vi "Esercitazione 4 - Incertezza di categoria A.vi"() -> ()   [LabVIEW 2021]
panel:
  out "Relative uncertainty value (%)":dbl
  out "Absolute uncertainty":dbl format="%#_6f"
  out "Experimental waste":dbl format="%#_6f"
  out "Array":dbl[](array[numeric])
  out "Best estimate of the measurand":dbl
  out "sum":dbl
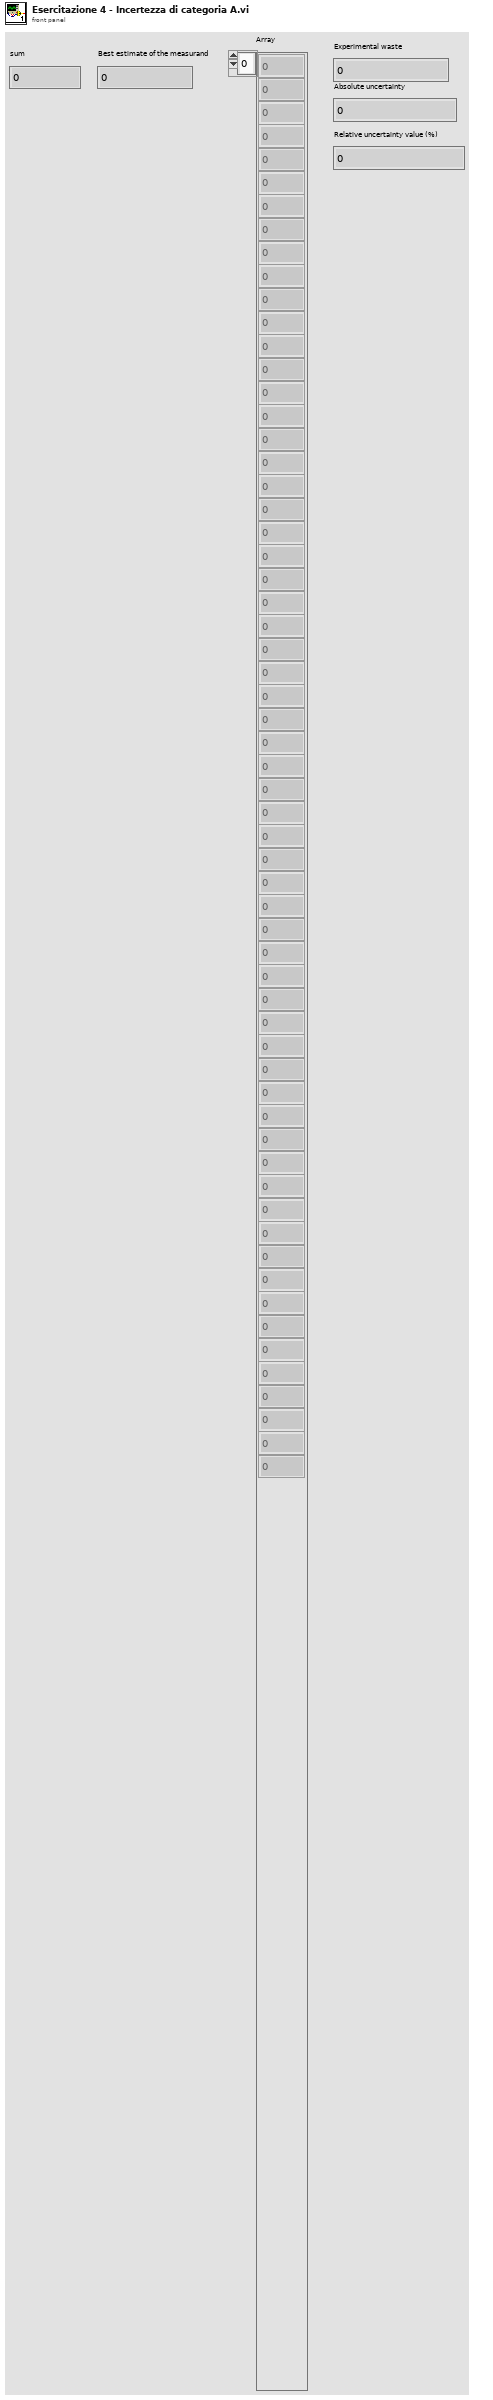
[diagram p1: front panel]
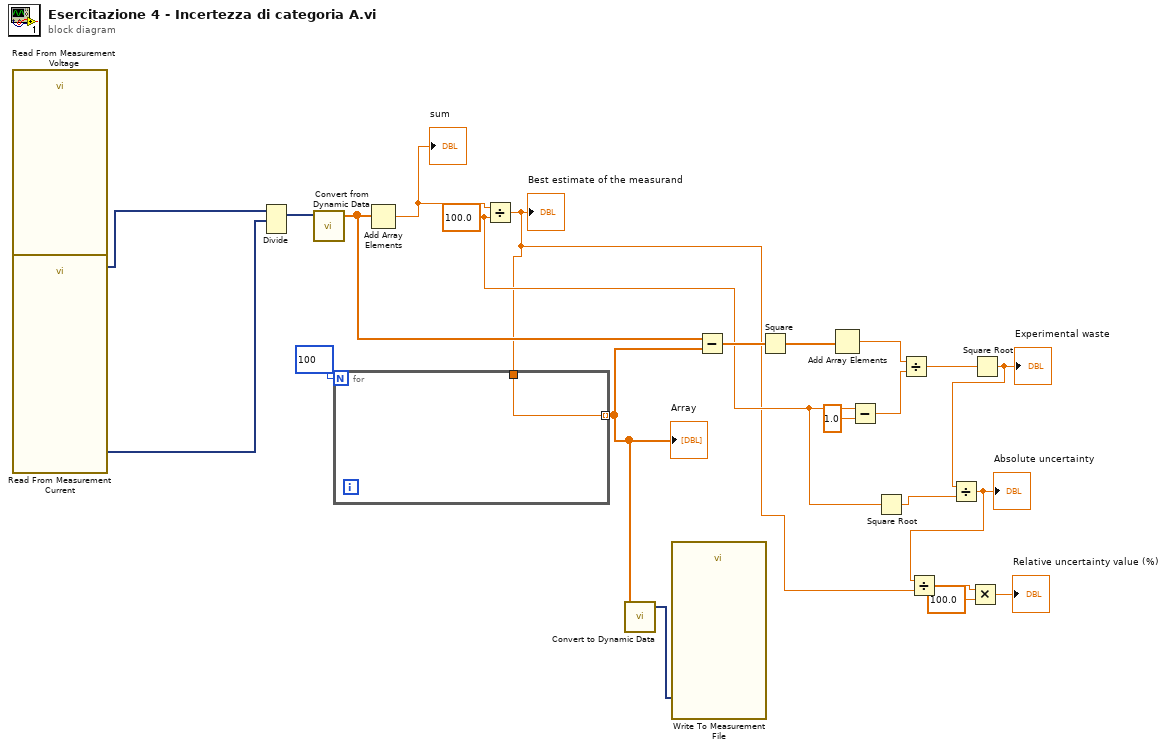
[diagram p0: block diagram]
diagram:
  w7 = 100.0 ("y")
  n1 = call "Read From Measurement Voltage"() -> ("Signals"=w22:dynamicdata)  [unwired: 6 in, 5 out]
  n2 = call "Read From Measurement Current"() -> ("Signals"=w21:dynamicdata)  [unwired: 6 in, 5 out]
  n3 = Divide(1:w21, 2:w22) -> (0:w1:dynamicdata)  [unwired: 1 in, 1 out]
  n4 = call "Convert from Dynamic Data"("Dynamic Data Type"=w1) -> ("Array"=w15:dbl[])  [unwired: 3 in]
  n5 = Add Array Elements(numeric array=w15) -> (sum=w20:dbl)
  "sum" <- w20
  n6 = Divide(x=w20, y=w7) -> (x/y=w5:dbl)
  "Best estimate of the measurand" <- w5
  n7 = for {
    N: 100 -> [_]
    tunnel: w5 -> [w23]
    tunnel: [w23] -> w18 mode=indexing
  }
  "Array" <- w18
  n8 = call "Convert to Dynamic Data"("Array"=w18) -> ("Dynamic Data Type"=w17:dynamicdata)  [unwired: 3 in]
  n9 = call "Write To Measurement File"("Signals"=w17) -> ()  [unwired: 16 in, 3 out]
  n10 = Subtract(x=w15, y=w18) -> (x-y=w16:dbl[])
  n11 = Square(x=w16) -> (x^2=w14:dbl[])
  n12 = Add Array Elements(numeric array=w14) -> (sum=w13:dbl)
  n13 = Subtract(x=w7, y=1.0) -> (x-y=w10:dbl)
  n14 = Square Root(x=w7) -> (sqrt(x)=w8:dbl)
  n15 = Divide(x=w13, y=w10) -> (x/y=w12:dbl)
  n16 = Square Root(x=w12) -> (sqrt(x)=w11:dbl)
  "Experimental waste" <- w11
  n17 = Divide(x=w11, y=w8) -> (x/y=w6:dbl)
  "Absolute uncertainty" <- w6
  n18 = Divide(x=w6, y=w5) -> (x/y=w4:dbl)
  n19 = Multiply(x=w4, y=100.0) -> (x*y=→"Relative uncertainty value (%)":dbl)
